vi "Write Triggers to TDMS.vi"(9 "Triggers":cluster{dbl[], dbl[]}[](array[cluster]), 10 "Layer #":i32, 11 "Refnum in":refnum<k34>) -> (3 "Refnum out":refnum<k34>)   [LabVIEW 2016]
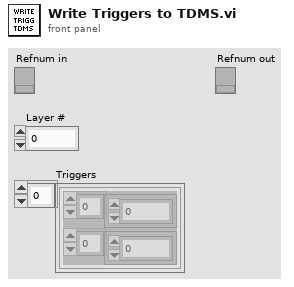
[diagram p1: front panel]
types:
  T1 = cluster{"Triggers[0]":cluster{dbl[], dbl[]}, "Triggers[1]":cluster{dbl[], dbl[]}, "Triggers[2]":cluster{dbl[], dbl[]}, "Triggers[3]":cluster{dbl[], dbl[]}, "Triggers[4]":cluster{dbl[], dbl[]}}
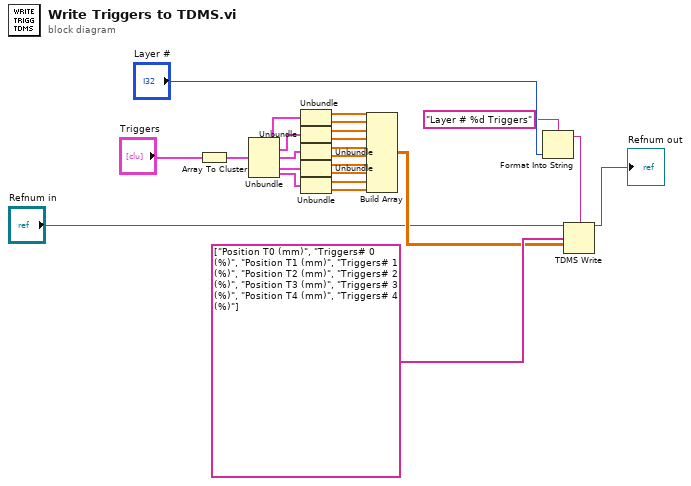
[diagram p0: block diagram]
diagram:
  n1 = Array To Cluster(array="Triggers") -> (cluster=w15:T1)
  n2 = Unbundle(w15) -> ("Triggers[0]"=w16:cluster{dbl[], dbl[]}, "Triggers[1]"=w17:cluster{dbl[], dbl[]}, "Triggers[2]"=w18:cluster{dbl[], dbl[]}, "Triggers[3]"=w19:cluster{dbl[], dbl[]}, "Triggers[4]"=w20:cluster{dbl[], dbl[]})
  n3 = Unbundle(w16) -> (w21:dbl[], w9:dbl[])
  n4 = Unbundle(w17) -> (w8:dbl[], w7:dbl[])
  n5 = Unbundle(w18) -> (w6:dbl[], w5:dbl[])
  n6 = Unbundle(w19) -> (w4:dbl[], w3:dbl[])
  n7 = Unbundle(w20) -> (w2:dbl[], w1:dbl[])
  n8 = Build Array(w21, w9, w8, w7, w6, w5, w4, w3, w2, w1) -> (w22:dbl[][])
  n9 = Format Into String(format string="Layer # %d Triggers", "Layer #") -> (resulting string=w10:string)  [unwired: 2 in, 1 out]
  n10 = TDMS Write(0:"Refnum in", 5:w10, 7:string[] ["Position T0 (mm)", "Triggers# 0 (%)", "Position T1 (mm)", "Triggers# 1 (%)", "Position T2 (mm)", "Triggers# 2 (%)", "Position T3 (mm)", "Triggers# 3 (%)", "Position T4 (mm)", "Triggers# 4 (%)"] ("channel name(s) in (Untitled)"), 9:w22) -> (4:→"Refnum out":refnum<k34>)  [unwired: 2 in, 3 out]
